vi "Update GPIO Bank Output.vi"(0 "gpio bank":T1, 1 "gpio bank serdes id":T2, 11 "gpio bank output enable":T1) -> (4 "serdes id valid":bool)   [LabVIEW 2020, in "GettingStarted_Common_148X_FPGA.lvlib"]
uses:
  GettingStarted_Common_148X_FPGA.lvlib
  Types/SerDes Identifier.ctl
  <instrlib>/FlexRIO/CSI-2/v2/FPGA/Types/GPIO Bank.ctl
  <instrlib>/FlexRIO/CSI-2/v2/FPGA/NI CSI-2 API FPGA v2.lvlib
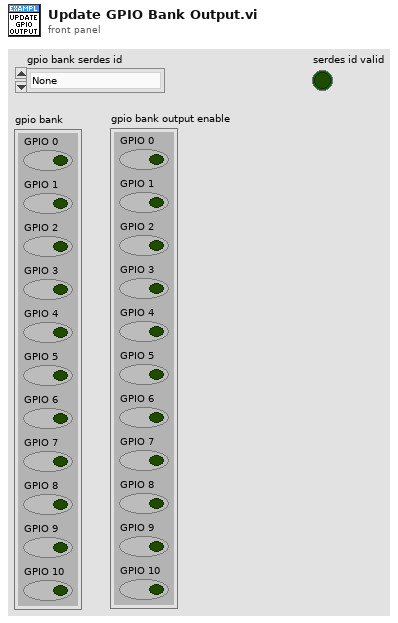
[diagram p1: front panel]
types:
  T1 = typedef "NI CSI-2 API FPGA v2.lvlib/GPIO Bank.ctl" = cluster{"GPIO 0":bool, "GPIO 1":bool, "GPIO 2":bool, "GPIO 3":bool, "GPIO 4":bool, "GPIO 5":bool, "GPIO 6":bool, "GPIO 7":bool, "GPIO 8":bool, "GPIO 9":bool, "GPIO 10":bool}
  T2 = typedef "GettingStarted_Common_148X_FPGA.lvlib/SerDes Identifier.ctl" = enum8{"None", "SI 0 Deserializer", "SI 1 Deserializer", "SI 2 Deserializer", "SI 3 Deserializer", "SI 4 Deserializer", "SI 5 Deserializer", "SI 6 Deserializer", "SI 7 Deserializer", "SO 0 Serializer", "SO 1 Serializer", "SO 2 Serializer", "SO 3 Serializer", "SO 4 Serializer", "SO 5 Serializer", "SO 6 Serializer", "SO 7 Serializer", "SI 0 SI 1 Deserializer", "SI 2 SI 3 Deserializer", "SI 4 SI 5 Deserializer", "SI 6 SI 7 Deserializer"}
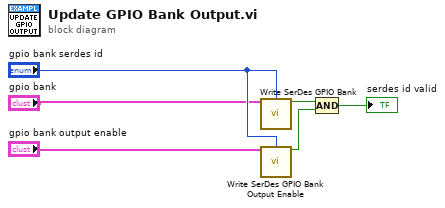
[diagram p0: block diagram]
diagram:
  n1 = call "Write SerDes GPIO Bank.vi"("gpio bank output"="gpio bank", "serdes id"="gpio bank serdes id") -> ("serdes id valid"=w2:bool)  [unwired: 13 in]
  n2 = call "Write SerDes GPIO Bank Output Enable.vi"("gpio bank output enable"="gpio bank output enable", "serdes id"="gpio bank serdes id") -> ("serdes id valid"=w3:bool)  [unwired: 13 in]
  n3 = Compound Arithmetic op=AND(w2, w3) -> (→"serdes id valid":bool)
